vi "GetProcessMode.vi"(8 "error in":errorcluster, 11 "ProcessRun in":refnum<class "ProcessRun.lvclass">) -> (0 "error out":errorcluster, 2 "ProcessMode":string, 3 "ProcessRun out":refnum<class "ProcessRun.lvclass">)   [LabVIEW 2021, in "ProligentXMLGenerator.lvlib" / "ProcessRun.lvclass"]
doc: "Defines the mode on which the process run has been ran, E.G. NPI, Production, etc.\n\nNon empty string restricted to 64 chars."
uses:
  ProcessRun.lvclass
  ProcessRun.lvclass/ProcessRun.ctl
  Base/NonEmptyString_64/NonEmptyString_64.lvclass
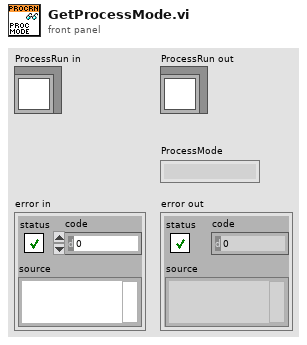
[diagram p1: front panel]
types:
  T1 = typedef "ProligentXMLGenerator.lvlib/ProcessRun.lvclass/Data.ctl" = cluster{"Name":string, "OperationRuns":refnum<class "OperationRun.lvclass">[], "OperationCycles":refnum<class "OperationCycle.lvclass">[], "FailureReferences":refnum<class "FailureReference.lvclass">[], "CustomData":refnum<class "CustomData.lvclass">, "ProcessRunId":refnum<class "Guid.lvclass">, "ProcessFullName":refnum<class "ProcessFullName.lvclass">, "ProcessVersion":refnum<class "NonEmptyString_64.lvclass">, "ProductUnitIdentifier":refnum<class "NonEmptyString_50.lvclass">, "ProductFullName":refnum<class "FullName.lvclass">, "ProcessRunStatus":refnum<class "ExecutionStatus.lvclass">, "ProcessRunStartTime":refnum<class "DateTime.lvclass">, "ProcessRunEndTime":refnum<class "DateTime.lvclass">, "ProcessMode":refnum<class "NonEmptyString_64.lvclass">, "TimeZoneInfoId":string}
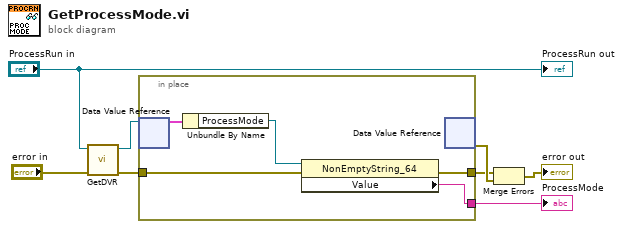
[diagram p0: block diagram]
diagram:
  n1 = call "GetDVR.vi"("error in"="error in", "ProcessRun"="ProcessRun in") -> ("error out"=w2:errorcluster, "DVRReference"=w7:refnum<data-value>)  [unwired: 8 in]
  n2 = in-place "In Place Element Structure" {
    in-place-border: [w10] -> w6
    in-place-border: w2 -> [w11]
    in-place-border: [w9] -> w1
    n3 = in-place-dvr #1(w7) -> (w13:T1)  [unwired: 1 out]
    n4 = Unbundle By Name(w13) -> ("ProcessMode"=w12:refnum<class "NonEmptyString_64.lvclass">)
    n5 = property on="Property Node" class="NonEmptyString_64"(reference=w12, error in=w11) -> (error out=w9:errorcluster, "Value"=w10:string)  [unwired: 1 out]
    n6 = in-place-dvr #1() -> (w8:errorcluster)  [unwired: 1 in, 1 out]
  }
  "ProcessMode" <- w6
  n7 = Merge Errors(w1, w8) -> (→"error out":errorcluster)
  "ProcessRun out" <- "ProcessRun in"
